vi "XIPIN_Partial_Reconfiguration_Decoupler_1_0.vi"   [LabVIEW 2017]
doc: "The Partial Reconfiguration Decoupler is used to maintain a stable Static/RP boundary during partial reconfiguration\n------------------------------------\n<b>Need License</b> : No"
uses:
  <vilib>/rvi/XilinxIP/XIPIN_XNode/niFpgaXIPIN.xnode
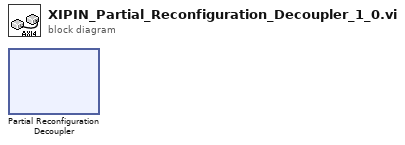
[diagram p0: block diagram]
diagram:
  n1 = xnode ("Partial Reconfiguration Decoupler")() -> ()
